vi "Container To String Docs.vi"() -> ()   [LabVIEW 2015]
uses:
  <vilib>/measure/NI_MABase.lvlib
panel:
  out "string":string
  out "string":string
  out "string":string
  out "string":string
  out "string":string
  out "string":string
  out "string":string
  out "string":string
  out "string":string
  out "string":string
  out "string":string
  out "string":string
  out "string":string
  out "string":string
  out "string":string
  out "string":string
  out "string":string
  out "string":string
  out "string":string
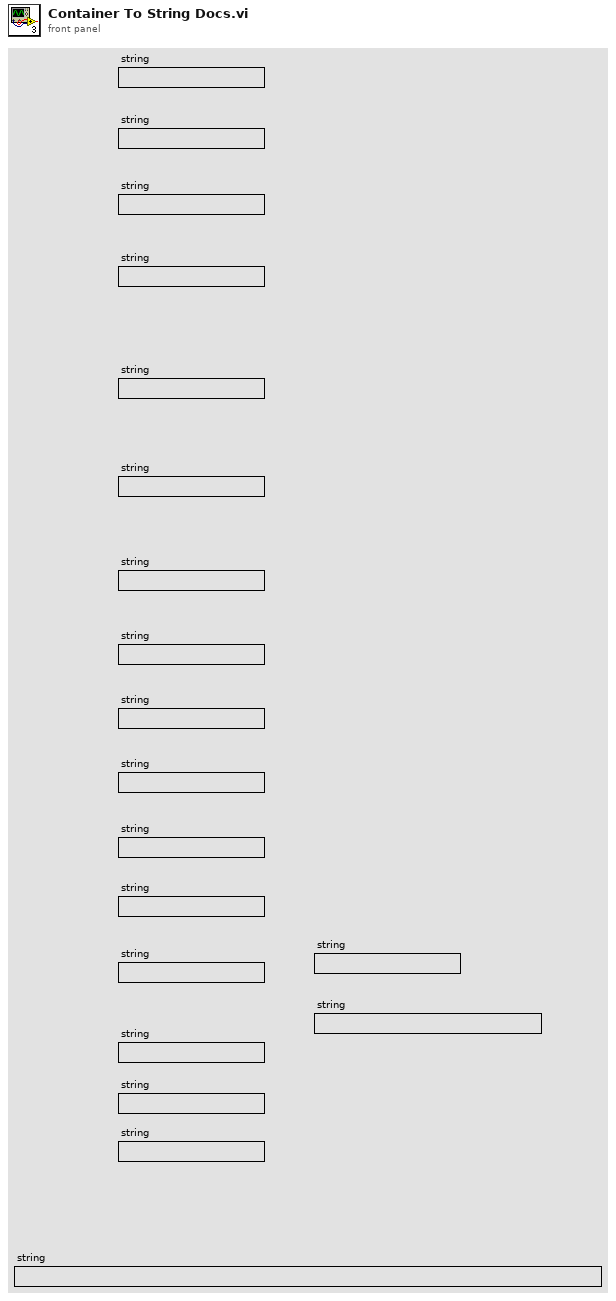
[diagram p1: front panel]
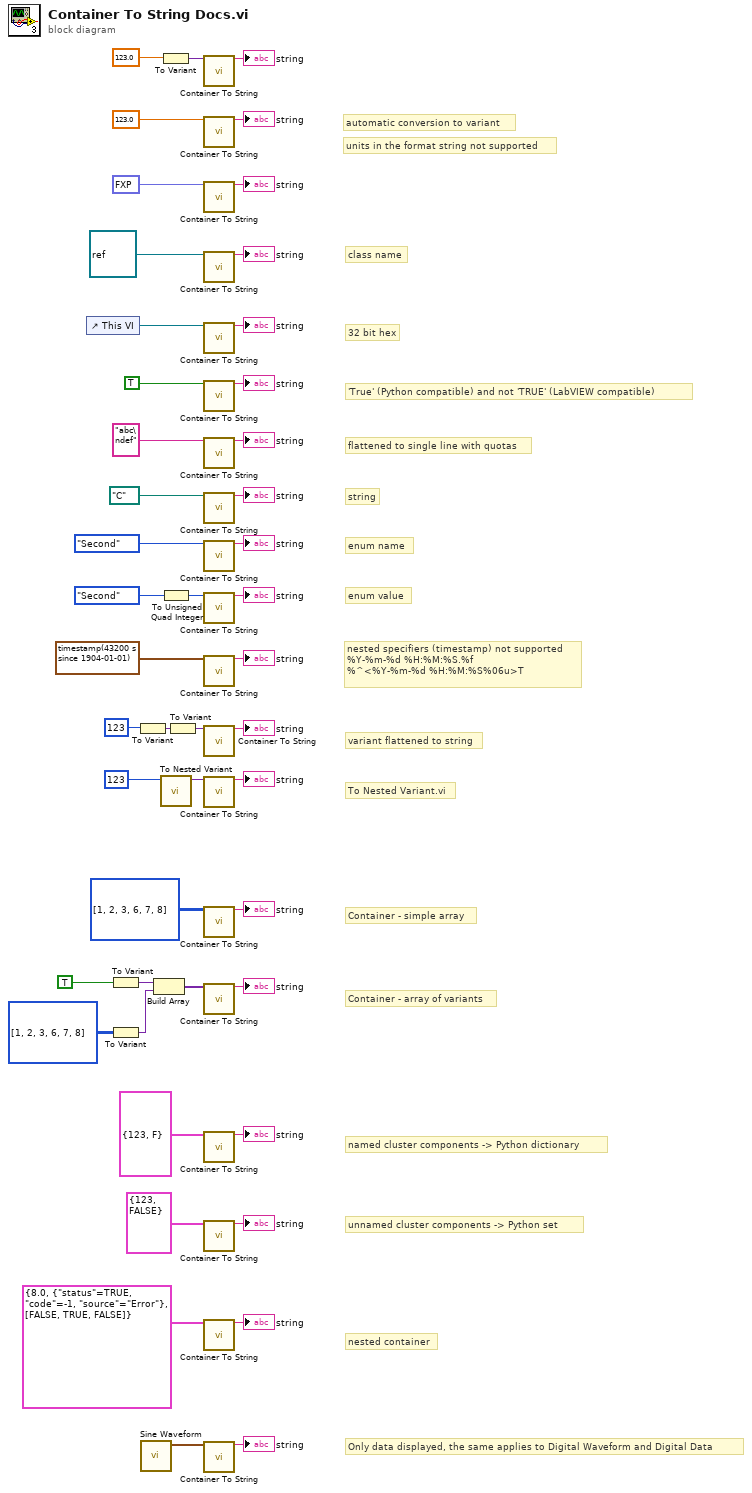
[diagram p0: block diagram]
diagram:
  # "nested container"
  # "Only data displayed, the same applies to Digital Waveform and Digital Data"
  # "Container - array of variants"
  # "Container - simple array"
  # "To Nested Variant.vi"
  # "variant flattened to string"
  # "nested specifiers (timestamp) not supported\n%Y-%m-%d %H:%M:%S.%f\n%^<%Y-%m-%d %H:%M:%S%06u>T"
  # "enum value"
  # "enum name"
  # "flattened to single line with quotas"
  # "string"
  # "'True' (Python compatible) and not 'TRUE' (LabVIEW compatible)"
  # "32 bit hex"
  # "class name"
  # "unnamed cluster components -> Python set"
  # "named cluster components -> Python dictionary"
  # "automatic conversion to variant"
  # "units in the format string not supported"
  n1 = control-ref of="This VI"() -> (w26:refnum<vi>)
  n2 = To Variant(anything=TRUE) -> (Variant=w43:variant)
  n3 = To Variant(anything=i32[][] [[1, 2, 3], [6, 7, 8]]) -> (Variant=w41:variant)
  n4 = To Variant(anything=123) -> (Variant=w45:variant)
  n5 = call <vilib>:"Sine Waveform.vi"() -> ("signal out"=w5:waveform(dbl))  [unwired: 10 in, 1 out]
  n6 = Build Array(w43, w41) -> (w12:variant[])
  n7 = To Variant(anything=123.0) -> (Variant=w40:variant)
  n8 = To Unsigned Quad Integer(1:enum16{"First", "Second"}."Second") -> (0:w6:u64)
  n9 = call "To Nested Variant.vi"("variant in"=123) -> ("variant out"=w9:variant)  [unwired: 10 in]
  n10 = To Variant(anything=w45) -> (Variant=w14:variant)
  n11 = call "Container To String.vi"("variant"=w40) -> ("string"=→"string":string)  [unwired: 12 in, 2 out]
  n12 = call "Container To String.vi"("variant"=123.0) -> ("string"=→"string":string)  [unwired: 12 in, 2 out]
  n13 = call "Container To String.vi"("variant"=fxp<+,4,2> 3.75) -> ("string"=→"string":string)  [unwired: 12 in, 2 out]
  n14 = call "Container To String.vi"("variant"=refnum<class> refnum ("object")) -> ("string"=→"string":string)  [unwired: 12 in, 2 out]
  n15 = call "Container To String.vi"("variant"=w26) -> ("string"=→"string":string)  [unwired: 12 in, 2 out]
  n16 = call "Container To String.vi"("variant"=TRUE) -> ("string"=→"string":string)  [unwired: 12 in, 2 out]
  n17 = call "Container To String.vi"("variant"="abc\ndef") -> ("string"=→"string":string)  [unwired: 12 in, 2 out]
  n18 = call "Container To String.vi"("variant"=path "C:/") -> ("string"=→"string":string)  [unwired: 12 in, 2 out]
  n19 = call "Container To String.vi"("variant"=enum16{"First", "Second"}."Second") -> ("string"=→"string":string)  [unwired: 12 in, 2 out]
  n20 = call "Container To String.vi"("variant"=w6) -> ("string"=→"string":string)  [unwired: 12 in, 2 out]
  n21 = call "Container To String.vi"("variant"=timestamp(43200 s since 1904-01-01) ("Time Stamp")) -> ("string"=→"string":string)  [unwired: 12 in, 2 out]
  n22 = call "Container To String.vi"("variant"=w14) -> ("string"=→"string":string)  [unwired: 12 in, 2 out]
  n23 = call "Container To String.vi"("variant"=w9) -> ("string"=→"string":string)  [unwired: 12 in, 2 out]
  n24 = call "Container To String.vi"("variant"=i32[][] [[1, 2, 3], [6, 7, 8]]) -> ("string"=→"string":string)  [unwired: 12 in, 2 out]
  n25 = call "Container To String.vi"("variant"=w12) -> ("string"=→"string":string)  [unwired: 12 in, 2 out]
  n26 = call "Container To String.vi"("variant"=cluster{"foo":i32, "bar":bool} {"foo"=123, "bar"=FALSE}) -> ("string"=→"string":string)  [unwired: 12 in, 2 out]
  n27 = call "Container To String.vi"("variant"=cluster{i32, bool} {123, FALSE}) -> ("string"=→"string":string)  [unwired: 12 in, 2 out]
  n28 = call "Container To String.vi"("variant"=cluster{dbl, errorcluster, bool[]} {8.0, {"status"=TRUE, "code"=-1, "source"="Error"}, [FALSE, TRUE, FALSE]}) -> ("string"=→"string":string)  [unwired: 12 in, 2 out]
  n29 = call "Container To String.vi"("variant"=w5) -> ("string"=→"string":string)  [unwired: 12 in, 2 out]
